vi "QCA Check Baseline.vi"(2 "error in (no error)":errorcluster, 3 "event number":i32, 4 "modulation (kHz)":i32, 5 "frequency (MHz)":dbl) -> (0 "error out":errorcluster, 1 "match?":bool)   [LabVIEW 2010]
uses:
  TCL-Target_Computer_Logging/TCL Get Base Fragments/TCL Get Base Fragments - 1eventNfrag.vi
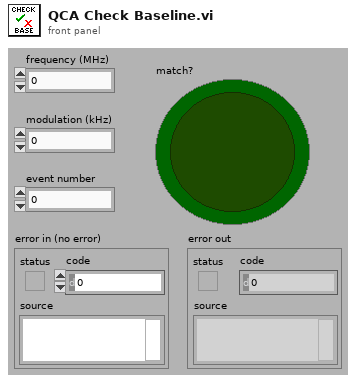
[diagram p1: front panel]
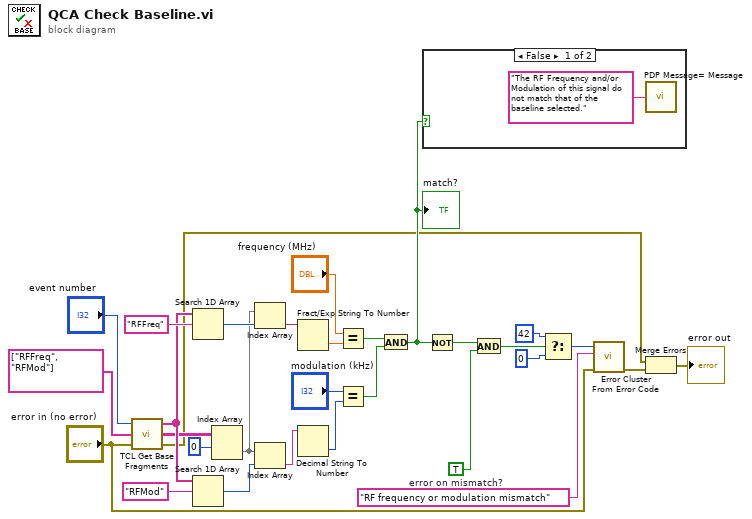
[diagram p0: block diagram]
diagram:
  w10 = TRUE  # error on mismatch?
  n1 = call-poly "TCL Get Base Fragments.vi"("error in (no error)"="error in (no error)", "fragments"=string[] ["RFFreq", "RFMod"] ("fragment"), "event number"="event number") -> ("error out"=w1:errorcluster, "values"=w20:string[][], "fragments out"=w23:string[])
  n2 = Search 1D Array(1D array=w23, element="RFFreq") -> (index of element=w27:i32)  [unwired: 1 in]
  n3 = Search 1D Array(1D array=w23, element="RFMod") -> (index of element=w21:i32)  [unwired: 1 in]
  n4 = Index Array(array=w20, index (row)=0) -> (element=w18:string[])  [unwired: 1 in]
  n5 = Index Array(array=w18, index=w27) -> (element=w26:string)
  n6 = Index Array(array=w18, index=w21) -> (element=w17:string)
  n7 = Fract/Exp String To Number(string=w26) -> (number=w25:dbl)  [unwired: 3 in, 1 out]
  n8 = Decimal String To Number(string=w17) -> (number=w15:i32)  [unwired: 2 in, 1 out]
  n9 = Equal?(x="frequency (MHz)", y=w25) -> (x = y?=w14:bool)
  n10 = Equal?(x="modulation (kHz)", y=w15) -> (x = y?=w13:bool)
  n11 = And(x=w14, y=w13) -> (x .and. y?=w12:bool)
  "match?" <- w12
  n12 = case shown="False" w12 {
    frame False {
      n13 = call "PDP Message= Message.vi"("Message"="The RF Frequency and/or Modulation of this signal do not match that of the baseline selected.") -> ()
    }
    frame True {
    }
  }
  n14 = Not(x=w12) -> (.not. x?=w11:bool)
  n15 = And(x=w11, y=w10) -> (x .and. y?=w8:bool)
  n16 = Select(t=42, s=w8, f=0) -> (s? t:f=w5:i32)
  n17 = call <vilib>:"Error Cluster From Error Code.vi"("error in (no error)"="error in (no error)", "error message (\"\")"="RF frequency or modulation mismatch" ("error message (\"\")"), "error code (0)"=w5) -> ("error out"=w3:errorcluster)  [unwired: 6 in]
  n18 = Merge Errors(w1, w3) -> (→"error out":errorcluster)
